vi "find all com ports.vi"() -> (3 "com ports array":string[](array[string]))   [LabVIEW 2017]
doc: "SciScan 1.2 160622"
panel:
  out "error out":errorcluster
  out "find list":string[](array[string])
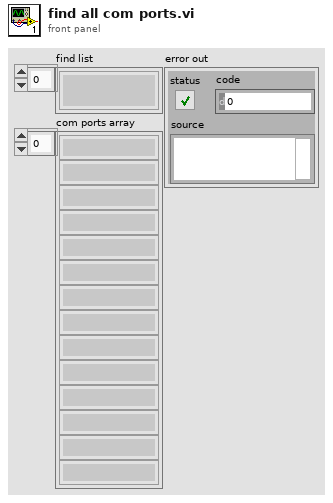
[diagram p1: front panel]
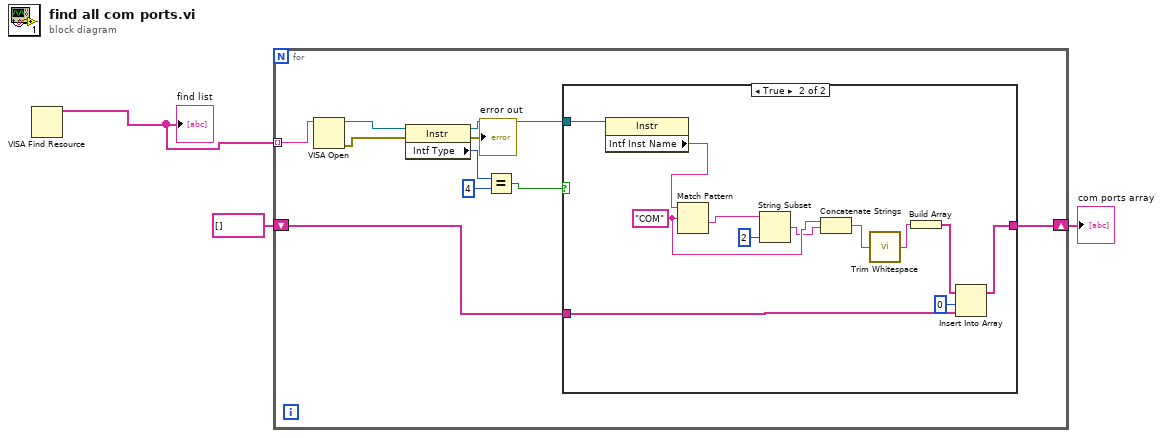
[diagram p0: block diagram]
diagram:
  n1 = VISA Find Resource() -> (3:w3:string[])  [unwired: 3 in, 2 out]
  "find list" <- w3
  n2 = for {
    tunnel: w3 -> [w13] mode=indexing
    shift-right: [w7] -> w1
    shift-left: string[] [] -> [w6]
    n3 = VISA Open(VISA resource name=w13) -> (VISA resource name=w12:refnum<visa-resource-name>, error out=w5:errorcluster)  [unwired: 4 in]
    n4 = property class="Instr"(reference=w12, error in=w5) -> (reference out=w9:refnum<visa-resource-name>, error out=→"error out":errorcluster, "Intf Type"=w11:u16)
    n5 = Equal?(x=w11, y=u16 4) -> (x = y?=w8:bool)
    n6 = case shown="True" w8 {
      tunnel: w9 -> [_ w26]
      tunnel: [w14 w17] -> w7
      tunnel: w6 -> [w14 w19]
      frame False {
      }
      frame True {
        w22 = "COM" ("regular expression")
        n7 = property class="Instr"(reference=w26) -> ("Intf Inst Name"=w25:string)  [unwired: 1 in, 2 out]
        n8 = Match Pattern(string=w25, regular expression=w22) -> (after substring=w24:string)  [unwired: 1 in, 3 out]
        n9 = String Subset(string=w24, length (rest)=2 ("length (rest)")) -> (substring=w21:string)  [unwired: 1 in]
        n10 = Concatenate Strings(w22, w21) -> (w16:string)
        n11 = call <vilib>:"Trim Whitespace.vi"("string"=w16) -> ("trimmed string"=w15:string)  [unwired: 1 in]
        n12 = Build Array(w15) -> (w20:string[])
        n13 = Insert Into Array(array=w20, index=0, new element=w19) -> (w17:string[])
      }
    }
  }
  "com ports array" <- w1
